vi "VerifyCertificates.vi"(7 "server url":string, 8 "error in (no error)":errorcluster, 9 "SSL ref":i32, 10 "NIssleay path":path, 11 "NIlibeay path":path) -> (0 "error out":errorcluster)   [LabVIEW 2015]
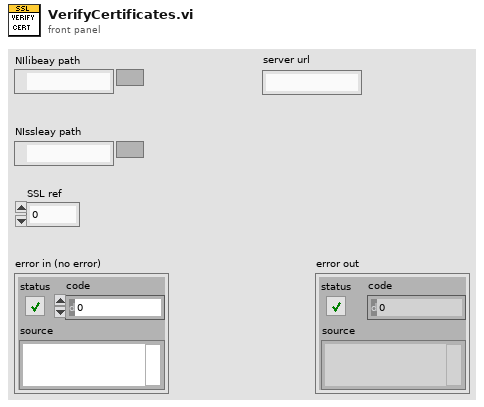
[diagram p1: front panel]
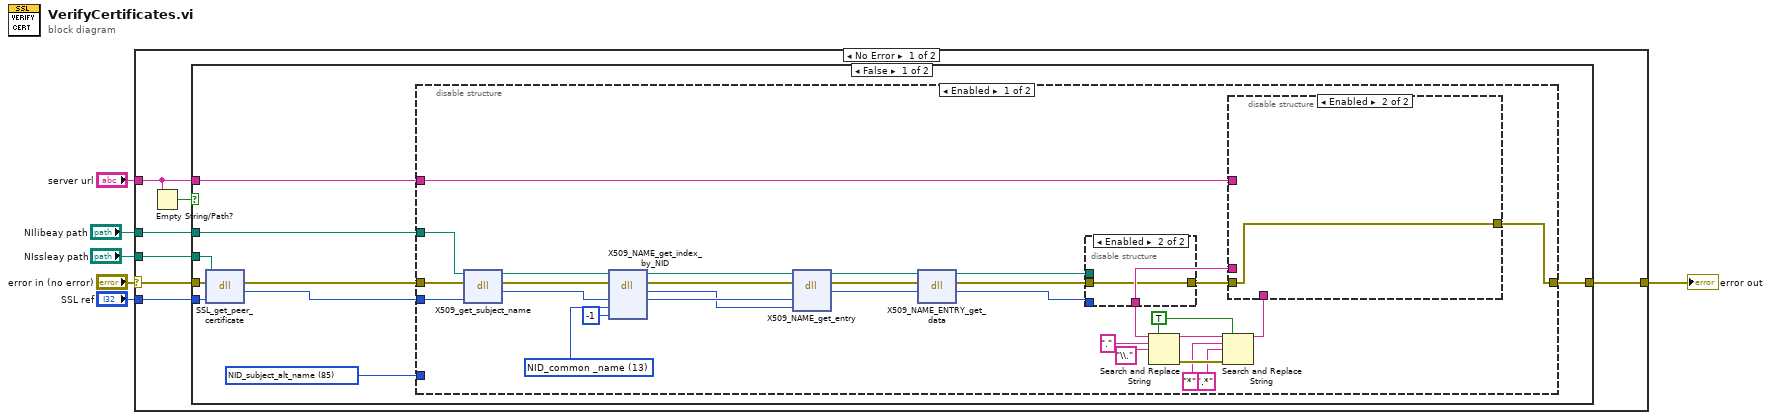
[diagram p0: block diagram]
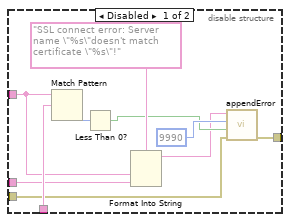
[diagram p2: hidden frame]
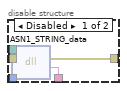
[diagram p3: hidden frame]
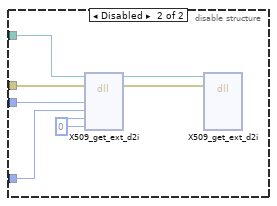
[diagram p4: hidden frame]
diagram:
  n1 = case shown="No Error" "error in (no error)" {
    selector: "error in (no error)" -> [w10 w78]
    tunnel: "SSL ref" -> [w13 _]
    tunnel: "NIlibeay path" -> [w12 _]
    tunnel: [w11 w78] -> w3
    tunnel: "server url" -> [w9 _]
    tunnel: "NIssleay path" -> [w7 _]
    frame No Error {
      n2 = Empty String/Path?(string/path=w9) -> (empty?=w8:bool)
      n3 = case shown="False" w8 {
        tunnel: w13 -> [w20 _]
        tunnel: w12 -> [w19 _]
        tunnel: [w17 w77] -> w11
        tunnel: w9 -> [w16 _]
        tunnel: w10 -> [w15 w77]
        tunnel: w7 -> [w14 _]
        frame False {
          w18 = 85 items=["NID_common _name"=13, "NID_subject_alt_name"=85]
          n4 = dll-call lib="NIssleay32.*" fn="SSL_get_peer_certificate"(path in=w14, error in=w15, "SSL"=w20) -> (error out=w22:errorcluster, "x509 pointer"=w21:i32)  [unwired: 2 in, 1 out]
          n5 = disable-structure shown="Enabled" {
            disable-tunnel: w22 -> [w37 w76]
            disable-tunnel: w21 -> [w36 w74]
            disable-tunnel: [w23 _] -> w17
            disable-tunnel: w19 -> [w35 w75]
            disable-tunnel: w18 -> [_ w73]
            disable-tunnel: w16 -> [w25 _]
            frame Enabled {
              w33 = TRUE ("replace all? (F)")
              w39 = 13 items=["NID_common _name"=13, "NID_subject_alt_name"=85]
              n6 = dll-call lib="NIlibeay32.*" fn="X509_get_subject_name"(path in=w35, error in=w37, "Server_Cert"=w36) -> (path out=w41:path, error out=w40:errorcluster, "X509 pointer"=w47:i32)  [unwired: 2 in]
              n7 = dll-call lib="NIlibeay32.*" fn="X509_NAME_get_index_by_NID"(path in=w41, error in=w40, "X509 cert"=w47, "NID-type"=w39, "start offset"=-1) -> (path out=w43:path, error out=w46:errorcluster, "location"=w44:i32, "X509 cert"=w45:i32)  [unwired: 3 in]
              n8 = dll-call lib="NIlibeay32.*" fn="X509_NAME_get_entry"(path in=w43, error in=w46, "X509 cert"=w45, "location"=w44) -> (path out=w42:path, error out=w48:errorcluster, "entry pointer"=w49:i32)  [unwired: 3 in]
              n9 = dll-call lib="NIlibeay32.*" fn="X509_NAME_ENTRY_get_data"(path in=w42, error in=w48, "entry pointer"=w49) -> (path out=w50:path, error out=w52:errorcluster, "ASN1 pointer"=w51:i32)  [unwired: 2 in]
              n10 = disable-structure shown="Enabled" {
                disable-tunnel: w52 -> [w68 w69]
                disable-tunnel: w51 -> [w67 _]
                disable-tunnel: w50 -> [w66 _]
                disable-tunnel: [w65 _] -> w26
                disable-tunnel: [w64 w69] -> w24
                frame Disabled {
                  n11 = dll-call lib="NIlibeay32.*" fn="ASN1_STRING_data"(path in=w66, error in=w68, "ASN1 pointer"=w67) -> (error out=w64:errorcluster, "string"=w65:string)  [unwired: 2 in, 1 out]
                }
                frame Enabled {
                }
              }
              n12 = Search and Replace String(replace all?=w33, input string=w26, search string=".", replace string="\\." ("search string")) -> (result string=w30:string, error out=w34:errorcluster)  [unwired: 4 in, 2 out]
              n13 = Search and Replace String(replace all?=w33, input string=w30, search string="*", replace string=".*" ("search string"), error in=w34) -> (result string=w27:string)  [unwired: 3 in, 3 out]
              n14 = disable-structure shown="Enabled" {
                disable-tunnel: w27 -> [w62 _]
                disable-tunnel: w26 -> [w60 _]
                disable-tunnel: w25 -> [w59 _]
                disable-tunnel: w24 -> [w57 w63]
                disable-tunnel: [w56 w63] -> w23
                frame Disabled {
                  n15 = Match Pattern(string=w59, regular expression=w62) -> (offset past match=w61:i32)  [unwired: 1 in, 3 out]
                  n16 = Less Than 0?(x=w61) -> (x < 0?=w54:bool)
                  n17 = Format Into String(format string="SSL connect error: Server name \"%s\"doesn't match certificate \"%s\"!" ("error message (\"\")"), w59, w60) -> (resulting string=w53:string)  [unwired: 2 in, 1 out]
                  n18 = call "appendError.vi"("error in (no error)"=w57, "Boolean"=w54, "code"=9990, "String"=w53) -> ("error out"=w56:errorcluster)  [unwired: 7 in]
                }
                frame Enabled {
                }
              }
            }
            frame Disabled {
              w72 = 0 ("arg3")
              n19 = dll-call lib="C:/Program Files (x86)/National Instruments/Shared/nissl/NIlibeay32.dll" fn="X509_get_ext_d2i"(path in=w75, error in=w76, "x509 pointer"=w74, "NID"=w73, "arg3"=w72, "arg4"=w72) -> (path out=w70:path, error out=w71:errorcluster)  [unwired: 6 in]
              n20 = dll-call lib="C:/Program Files (x86)/National Instruments/Shared/nissl/NIlibeay32.dll" fn="X509_get_ext_d2i"(path in=w70, error in=w71) -> ()  [unwired: 10 in, 2 out]
            }
          }
        }
        frame True {
        }
      }
    }
    frame Error {
    }
  }
  "error out" <- w3
